vi "EnumerateAndSortDevices.vi"(8 "error in (no error)":errorcluster) -> (0 "error out":errorcluster, 2 "Devices (ordered)":tag[](array[tag])=["PXI1Slot2", "PXI1Slot3", "PXI1Slot5", "PXI1Slot6", "PXI1Slot7", "PXI1Slot8"], 3 "Devices":T1(array[cluster]))   [LabVIEW 2019, in "Instrument.Lockin.lvlib" / "Instrument.DAQ.lvclass"]
uses:
  Instrument.DAQ.lvclass
  <resource>/objmgr/daqmx.rc
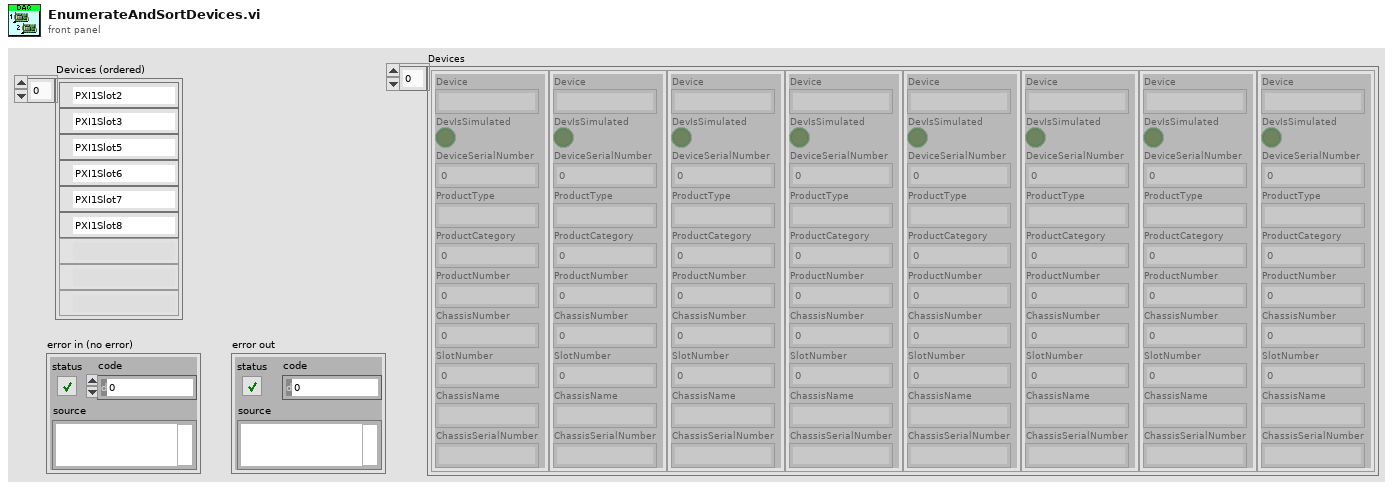
[diagram p1: front panel]
types:
  T1 = cluster{"Device":string, "DevIsSimulated":bool, "DeviceSerialNumber":u32, "ProductType":string, "ProductCategory":i32, "ProductNumber":u32, "ChassisNumber":u32, "SlotNumber":u32, "ChassisName":string, "ChassisSerialNumber":string}[]
  T2 = cluster{"Device":string, "DevIsSimulated":bool, "DeviceSerialNumber":u32, "ProductType":string, "ProductCategory":i32, "ProductNumber":u32, "ChassisNumber":u32, "SlotNumber":u32, "ChassisName":string, "ChassisSerialNumber":string}
  T3 = cluster{"Device":string, "DeviceSerialNumber":u32, "ProductType":string, "ProductCategory":i32, "ProductNumber":u32, "ChassisNumber":u32, "SlotNumber":u32, "ChassisName":string, "ChassisSerialNumber":string}
  T4 = cluster{"PxiChassisNumber":u32, "ProductName":string, "SerialNumber":string}[]
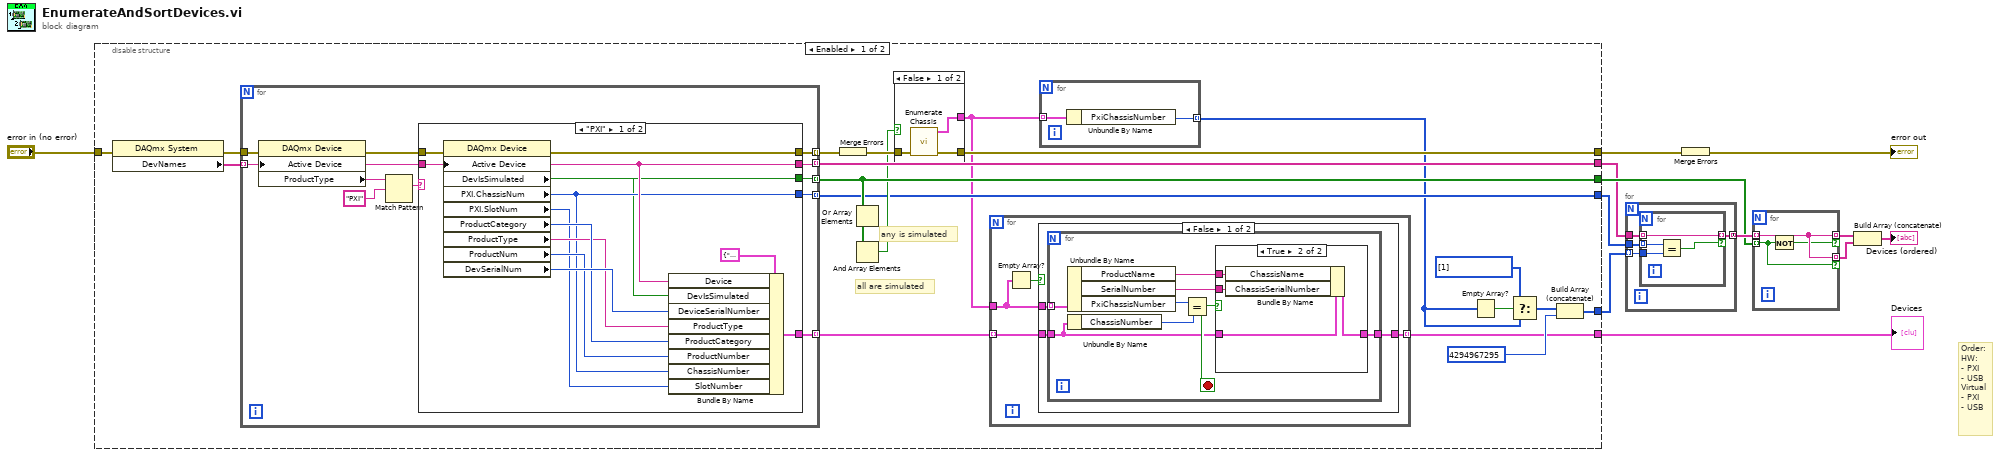
[diagram p0: block diagram]
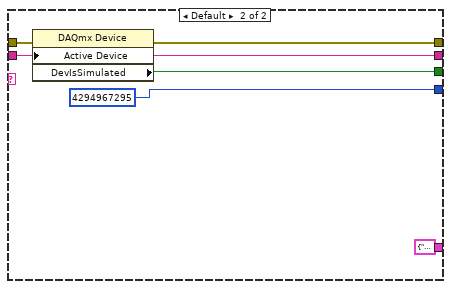
[diagram p2: hidden frame]
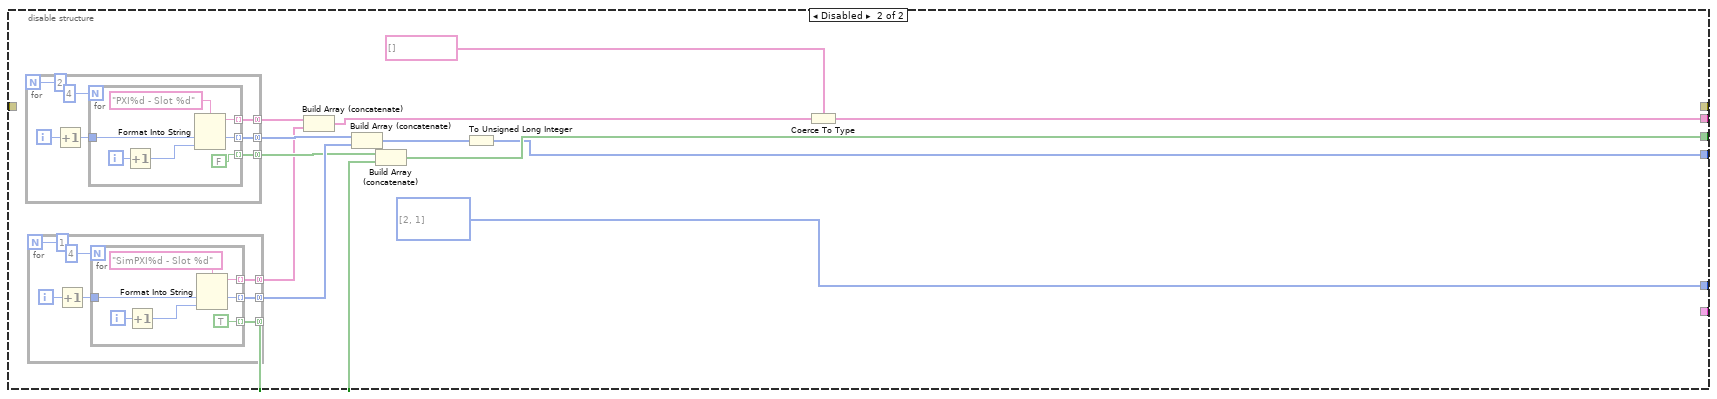
[diagram p6: hidden frame]
diagram:
  # "Order:\nHW:\n- PXI\n- USB\nVirtual\n- PXI\n- USB"
  n1 = disable-structure shown="Enabled" {
    disable-tunnel: "error in (no error)" -> [w20 _]
    disable-tunnel: [w21 _] -> w10
    disable-tunnel: [w27 u32[] [2, 1] ("PxiChassis Numbers")] -> w4
    disable-tunnel: [w31 w100] -> w2
    disable-tunnel: [w19 w88] -> w8
    disable-tunnel: [w17 w87] -> w3
    disable-tunnel: [w14 _] -> w1
    frame Enabled {
      # "all are simulated"
      # "any is simulated"
      n2 = property class="DAQmx System"(error in=w20) -> (error out=w30:errorcluster, "DevNames"=w29:tag[])  [unwired: 1 in, 1 out]
      n3 = for {
        tunnel: w29 -> [w34] mode=indexing
        tunnel: w30 -> [w42]
        tunnel: [w35] -> w23 mode=indexing
        tunnel: [w33] -> w31 mode=indexing
        tunnel: [w41] -> w19 mode=indexing
        tunnel: [w40] -> w17 mode=indexing
        tunnel: [w32] -> w15 mode=indexing
        n4 = property class="DAQmx Device"(error in=w42, "Active Device"=w34) -> (error out=w36:errorcluster, "ProductType"=w39:string)  [unwired: 1 in, 1 out]
        n5 = Match Pattern(string=w39, regular expression="PXI") -> (match substring=w38:string)  [unwired: 1 in, 3 out]
        n6 = case shown="\"PXI\"" w38 {
          tunnel: [w43 w59] -> w41
          tunnel: [w47 u32 4294967295 ("PXI.ChassisNum")] -> w40
          tunnel: w36 -> [w54 w57]
          tunnel: [w53 w58] -> w35
          tunnel: w34 -> [w52 w55]
          tunnel: [w52 w55] -> w33
          tunnel: [w45 _] -> w32
          frame "PXI" {
            n7 = property class="DAQmx Device"(error in=w54, "Active Device"=w52) -> (error out=w53:errorcluster, "DevIsSimulated"=w43:bool, "PXI.ChassisNum"=w47:u32, "PXI.SlotNum"=w46:u32, "ProductCategory"=w50:i32, "ProductType"=w48:string, "ProductNum"=w49:u32, "DevSerialNum"=w51:u32)  [unwired: 1 in, 1 out]
            n8 = Bundle By Name(cluster=T2 {"Device"="", "DevIsSimulated"=FALSE, "DeviceSerialNumber"=0, "ProductType"="", "ProductCategory"=0, "ProductNumber"=0, "ChassisNumber"=0, "SlotNumber"=0, "ChassisName"="", "ChassisSerialNumber"=""} ("output cluster"), "Device"=w52, "DevIsSimulated"=w43, "DeviceSerialNumber"=w51, "ProductType"=w48, "ProductCategory"=w50, "ProductNumber"=w49, "ChassisNumber"=w47, "SlotNumber"=w46) -> (w45:T2)
          }
          frame Default {
            (unwired) T3 {"Device"="", "DeviceSerialNumber"=0, "ProductType"="", "ProductCategory"=0, "ProductNumber"=0, "ChassisNumber"=0, "SlotNumber"=0, "ChassisName"="", "ChassisSerialNumber"=""} ("Cluster")
            n9 = property class="DAQmx Device"(error in=w57, "Active Device"=w55) -> (error out=w58:errorcluster, "DevIsSimulated"=w59:bool)  [unwired: 1 in, 1 out]
          }
        }
      }
      n10 = Merge Errors(w23) -> (w22:errorcluster)
      n11 = Or Array Elements(Boolean array=w19) -> ()  [unwired: 1 out]
      n12 = And Array Elements(Boolean array=w19) -> (logical AND=w18:bool)
      n13 = case shown="False" w18 {
        tunnel: w22 -> [w83 w84]
        tunnel: [w82 w84] -> w21
        tunnel: [w81 _] -> w16
        frame False {
          n14 = call "Enumerate Chassis.vi"("error in (no error)"=w83) -> ("error out"=w82:errorcluster, "Chassis"=w81:T4)  [unwired: 9 in]
        }
        frame True {
        }
      }
      n15 = for {
        tunnel: w16 -> [w61]
        tunnel: w15 -> [w62] mode=indexing
        tunnel: [w63] -> w14 mode=indexing
        n16 = Empty Array?(array=w61) -> (empty?=w60:bool)
        n17 = case shown="False" w60 {
          tunnel: [w66 w80] -> w63
          tunnel: w62 -> [w65 w80]
          tunnel: w61 -> [w64 _]
          frame False {
            n18 = for {
              tunnel: w65 -> [w67]
              tunnel: w64 -> [w74] mode=indexing
              tunnel: [w69] -> w66
              stop <- w68 stop-if-true
              n19 = Unbundle By Name(w74) -> ("ProductName"=w71:string, "SerialNumber"=w70:string, "PxiChassisNumber"=w73:u32)
              n20 = Unbundle By Name(w67) -> ("ChassisNumber"=w72:u32)
              n21 = Equal?(x=w73, y=w72) -> (x = y?=w68:bool)
              n22 = case shown="True" w68 {
                tunnel: w67 -> [w75 w79]
                tunnel: w71 -> [_ w78]
                tunnel: w70 -> [_ w77]
                tunnel: [w75 w76] -> w69
                frame False {
                }
                frame True {
                  n23 = Bundle By Name(cluster=w79, "ChassisName"=w78, "ChassisSerialNumber"=w77) -> (w76:T2)
                }
              }
            }
          }
          frame True {
          }
        }
      }
      n24 = for {
        tunnel: w16 -> [w86] mode=indexing
        tunnel: [w85] -> w13 mode=indexing
        n25 = Unbundle By Name(w86) -> ("PxiChassisNumber"=w85:u32)
      }
      n26 = Empty Array?(array=w13) -> (empty?=w26:bool)
      n27 = Select(t=u32[] [1], s=w26, f=w13) -> (s? t:f=w24:u32[])
      n28 = Build Array (concatenate)(w24, u32 4294967295 ("x")) -> (w27:u32[])
    }
    frame Disabled {
      n29 = for {
        N: 2 -> [_]
        tunnel: [w119] -> w94 mode=concatenating
        tunnel: [w117] -> w93 mode=concatenating
        tunnel: [w114] -> w92 mode=concatenating
        i -> [w116]
        n30 = Increment(x=w116) -> (x+1=w115:i32)
        n31 = for {
          N: 4 -> [_]
          tunnel: [w124] -> w119 mode=indexing
          tunnel: w115 -> [w122]
          tunnel: [w122] -> w117 mode=indexing
          tunnel: [FALSE] -> w114 mode=indexing
          i -> [w125]
          n32 = Increment(x=w125) -> (x+1=w121:i32)
          n33 = Format Into String(format string="PXI%d - Slot %d", w122, w121) -> (resulting string=w124:string)  [unwired: 2 in, 1 out]
        }
      }
      n34 = for {
        N: 1 -> [_]
        tunnel: [w102] -> w91 mode=concatenating
        tunnel: [w106] -> w96 mode=concatenating
        tunnel: [w103] -> w95 mode=concatenating
        i -> [w105]
        n35 = Increment(x=w105) -> (x+1=w104:i32)
        n36 = for {
          N: 4 -> [_]
          tunnel: [w112] -> w102 mode=indexing
          tunnel: w104 -> [w110]
          tunnel: [w110] -> w106 mode=indexing
          tunnel: [TRUE] -> w103 mode=indexing
          i -> [w113]
          n37 = Increment(x=w113) -> (x+1=w109:i32)
          n38 = Format Into String(format string="SimPXI%d - Slot %d", w110, w109) -> (resulting string=w112:string)  [unwired: 2 in, 1 out]
        }
      }
      n39 = Build Array (concatenate)(w94, w91) -> (w89:string[])
      n40 = Build Array (concatenate)(w93, w96) -> (w90:i32[])
      n41 = Build Array (concatenate)(w92, w95) -> (w88:bool[])
      n42 = To Unsigned Long Integer(number=w90) -> (unsigned 32bit integer=w87:u32[])
      n43 = Coerce To Type(0:w89, 1:tag[] []) -> (2:w100:tag[])
    }
  }
  "Devices" <- w1
  n44 = for {
    tunnel: w2 -> [w129]
    tunnel: w3 -> [w128]
    tunnel: [w127] -> w9 mode=concatenating
    tunnel: w4 -> [w126] mode=indexing
    n45 = for {
      tunnel: [w133] -> w127 mode=indexing if=w130
      tunnel: w129 -> [w133] mode=indexing
      tunnel: w128 -> [w132] mode=indexing
      tunnel: w126 -> [w131]
      n46 = Equal?(x=w132, y=w131) -> (x = y?=w130:bool)
    }
  }
  n47 = Merge Errors(w10) -> (→"error out":errorcluster)
  n48 = for {
    tunnel: [w136] -> w7 mode=indexing if=w135
    tunnel: w9 -> [w136] mode=indexing
    tunnel: [w136] -> w6 mode=indexing if=w134
    tunnel: w8 -> [w134] mode=indexing
    n49 = Not(x=w134) -> (.not. x?=w135:bool)
  }
  n50 = Build Array (concatenate)(w7, w6) -> (→"Devices (ordered)":tag[])
